vi "Open System.vi"(4 "Clear Previous Connections (False)":bool, 6 "ID Query (True)":bool=TRUE, 7 "IP Address":string, 8 "error in (no error)":errorcluster, 9 "Serial Configuration":T4={"Baud Rate"=9600, "Parity"=0, "Data Bits"=8, "Stop Bits"=10, "Flow Control"=0} {"Flow Control" items=["None", "XON/XOFF", "RTS/CTS", "XON/XOFF & RTS/CTS", "DTR/DSR", "XON/XOFF & DTR/DSR"]; "Stop Bits" items=["1.0"=10, "2.0"=20]; "Data Bits" items=["7"=7, "8"=8]; "Parity" items=["None", "Odd", "Even"]; "Baud Rate" items=["300"=300, "600"=600, "1200"=1200, "2400"=2400, "4800"=4800, "9600"=9600, "19200"=19200]}, 10 "Comms Layer":T2, 11 "VISA resource name":refnum<visa-resource-name>) -> (0 "error out":errorcluster, 1 "# of Instruments":i32, 2 "Serial Number(s)":string[](array[string]), 3 "Mercury Reference Out":T1, 5 "S/W Version(s)":string[](array[string]))   [LabVIEW 2018, in "Mercury iXX.lvlib" / "System.lvlib"]
doc: "Opens communication with a Mercury instrument on the chosen communication bus."
uses:
  System.lvlib
  Serial Settings.ctl
  Comms Transport Layer.ctl
  Mercury Reference.ctl
  Query Dynamic Reference.ctl
  Lookup Reference FGV Enum.ctl
  VISA Flush IO Buffer Mask.ctl
  Mercury iXX.lvlib
panel:
  in  "Reset (True)":bool=TRUE
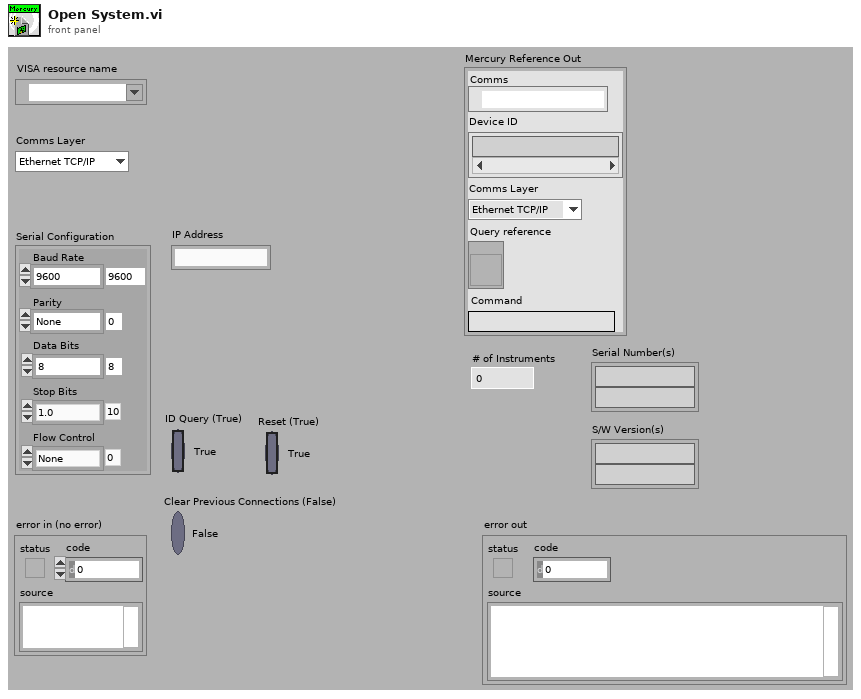
[diagram p1: front panel]
types:
  T1 = typedef "Mercury iXX.lvlib/Mercury Reference.ctl" = cluster{"Comms":refnum<visa-resource-name>, "Device ID":string[], "Comms Layer":T2, "Command":string, "Query reference":T3}
  T2 = typedef "Mercury iXX.lvlib/Comms Transport Layer.ctl" = enum16{"Ethernet TCP/IP", "USB", "ISOBus - RS-232", "GPIB"}
  T3 = typedef "Mercury iXX.lvlib/Query Dynamic Reference.ctl" = refnum<vi>
  T4 = typedef "Mercury iXX.lvlib/Serial Settings.ctl" = cluster{"Baud Rate":u32, "Parity":u16, "Data Bits":u16, "Stop Bits":u16, "Flow Control":u16}
  T5 = typedef "Mercury iXX.lvlib/Lookup Reference FGV Enum.ctl" = enum16{"Check VISA", "Get VI Ref", "Set VI ref", "Delete Single Ref", "Clear All"}
  T6 = typedef "VISA Flush IO Buffer Mask.ctl" = u16
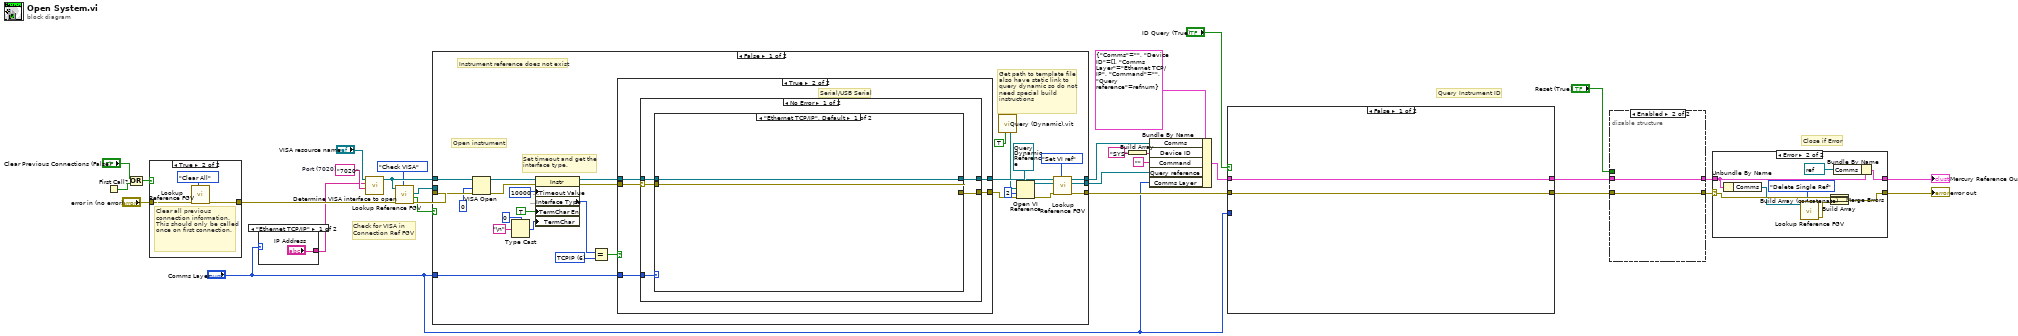
[diagram p0: block diagram]
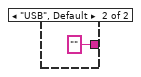
[diagram p2: hidden frame]
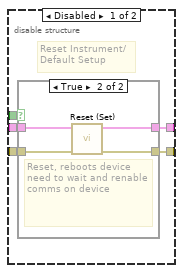
[diagram p4: hidden frame]
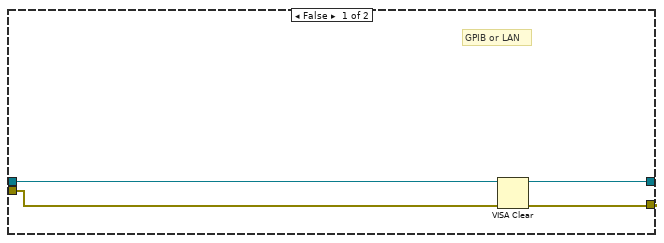
[diagram p6: hidden frame]
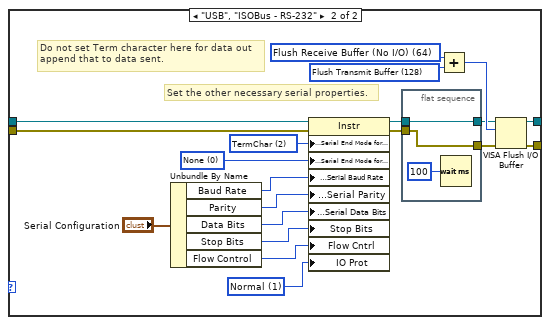
[diagram p7: hidden frame]
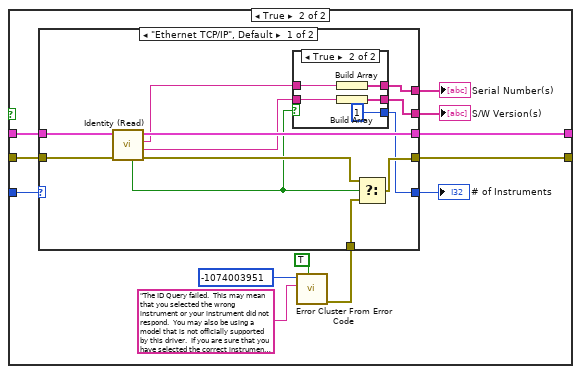
[diagram p11: hidden frame]
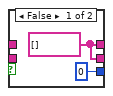
[diagram p12: hidden frame]
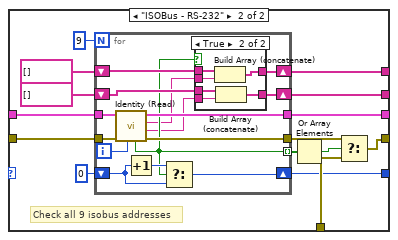
[diagram p13: hidden frame]
diagram:
  w30 = "7020"  # Port (7020)
  # "Check for VISA in \nConnection Ref FGV"
  # "Close if Error"
  # "Query Instrument ID"
  n1 = First Call?() -> (First Call?: T/F=w3:bool)
  n2 = Or(x="Clear Previous Connections (False)", y=w3) -> (x .or. y?=w4:bool)
  n3 = case shown="True" w4 {
    tunnel: "error in (no error)" -> [w31 w34]
    tunnel: [w31 w33] -> w5
    frame False {
    }
    frame True {
      # "Clear all previous connection information. This should only be called once on first connection."
      n4 = call "Lookup Reference FGV.vi"("State"=Lookup_Reference_FGV_Enum."Clear All", "error in"=w34) -> ("error out"=w33:errorcluster)  [unwired: 3 in, 6 out]
    }
  }
  n5 = case shown="\"Ethernet TCP/IP\"" "Comms Layer" {
    tunnel: ["IP Address" "" ("IP Address")] -> w1
    frame "Ethernet TCP/IP" {
    }
    frame "USB", Default {
    }
  }
  n6 = call "Determine VISA interface to open.vi"("Port (7020)"=w30, "IP Address"=w1, "VISA resource name"="VISA resource name") -> ("VISA resource name out"=w12:refnum<visa-resource-name>)  [unwired: 8 out]
  n7 = call "Lookup Reference FGV.vi"("State"=Lookup_Reference_FGV_Enum."Check VISA", "error in"=w5, "VISA In"=w12) -> ("error out"=w13:errorcluster, "Found Ref?"=w9:bool, "Query ref"=w8:T3)  [unwired: 2 in, 4 out]
  n8 = case shown="False" w9 {
    tunnel: w13 -> [w64 w108]
    tunnel: [w41 w108] -> w28
    tunnel: w12 -> [w54 w107]
    tunnel: [w43 w107] -> w16
    tunnel: "Comms Layer" -> [w49 _]
    tunnel: w8 -> [_ w106]
    tunnel: [w45 w106] -> w10
    frame False {
      w60 = u16 6 items=["GPIB"=1, "VXI"=2, "GPIB-VXI"=3, "Serial"=4, "PXI"=5, "TCPIP"=6, "USB"=7] ("Interface Information:Interface Type")
      # "Get path to template file\nalso have static link to \nquery dynamic so do not\nneed special build\ninstructions"
      # "Instrument reference does not exist"
      # "Set timeout and get the\ninterface type."
      # "Open instrument"
      n9 = VISA Open(access mode=u32 0, error in (no error)=w64, VISA resource name=w54) -> (VISA resource name=w58:refnum<visa-resource-name>, error out=w57:errorcluster)  [unwired: 2 out]
      n10 = Type Cast(type=u8 0 ("Message Based Settings:Termination Character"), x="\n") -> (*(type *) &x=w51:u8)
      n11 = property on="Property Node" class="Instr"(reference=w58, error in=w57, "General Settings:Timeout Value"=u32 10000, "TermChar En"=TRUE ("Message Based Settings:Termination Character Enable"), "TermChar"=w51) -> (reference out=w56:refnum<visa-resource-name>, error out=w55:errorcluster, "Interface Information:Interface Type"=w63:u16)
      n12 = Equal?(x=w63, y=w60) -> (x = y?=w61:bool)
      n13 = case shown="True" w61 {
        tunnel: [w66 w73] -> w44
        tunnel: [w65 w72] -> w47
        tunnel: w56 -> [w67 w71]
        tunnel: w55 -> [w68 w70]
        tunnel: w49 -> [_ w69]
        frame False {
          # "GPIB or LAN"
          n14 = VISA Clear(VISA resource name=w67, error in (no error)=w68) -> (VISA resource name out=w66:refnum<visa-resource-name>, error out=w65:errorcluster)
        }
        frame True {
          # "Serial/USB Serial"
          n15 = case shown="No Error" w70 {
            tunnel: w71 -> [w76 w105]
            selector: w70 -> [w75 w104]
            tunnel: [w78 w105] -> w73
            tunnel: [w77 w104] -> w72
            tunnel: w69 -> [w74 _]
            frame No Error {
              n16 = case shown="\"Ethernet TCP/IP\", Default" w74 {
                tunnel: [w80 w88] -> w78
                tunnel: [w79 w89] -> w77
                tunnel: w76 -> [w80 w90]
                tunnel: w75 -> [w79 w92]
                frame "Ethernet TCP/IP", Default {
                }
                frame "USB", "ISOBus - RS-232" {
                  w86 = T6 128 items=["Flush Receive Buffer"=16, "Write Transmit Buffer to Device"=32, "Flush Receive Buffer (No I/O)"=64, "Flush Transmit Buffer"=128] ("Mask")
                  w87 = T6 64 items=["Flush Receive Buffer"=16, "Write Transmit Buffer to Device"=32, "Flush Receive Buffer (No I/O)"=64, "Flush Transmit Buffer"=128] ("Mask")
                  w91 = u16 2 items=["None", "LastBit", "TermChar"] ("Serial Settings:Serial End Mode for Reads")
                  w100 = u16 1 items=["Normal"=1, "VXI/FDC"=2, "GPIB/HS488"=3, "Serial-TCPIP-USB/488 Strings"=4, "USBTMC/Vendor-Specific"=5] ("Message Based Settings:IO Protocol")
                  w95 = u16 0 items=["None", "LastBit", "TermChar"] ("Serial Settings:Serial End Mode for Reads")
                  # "Do not set Term character here for data out append that to data sent."
                  # "Set the other necessary serial properties."
                  n17 = Unbundle By Name("Serial Configuration") -> ("Baud Rate"=w97:u32, "Parity"=w99:u16, "Data Bits"=w98:u16, "Stop Bits"=w94:u16, "Flow Control"=w93:u16)
                  n18 = property on="Property Node" class="Instr"(reference=w90, error in=w92, "Serial Settings:Serial End Mode for Reads"=w91, "Serial Settings:Serial End Mode for Writes"=w95, "Serial Settings:Serial Baud Rate"=w97, "Serial Settings:Serial Parity"=w99, "Serial Settings:Serial Data Bits"=w98, "Stop Bits"=w94, "Flow Cntrl"=w93, "IO Prot"=w100) -> (reference out=w84:refnum<visa-resource-name>, error out=w82:errorcluster)
                  n19 = flat-sequence {
                    tunnel: w84 -> [w102]
                    tunnel: [w102] -> w83
                    tunnel: w82 -> [w101]
                    tunnel: [w101] -> w81
                    frame #0 {
                      n20 = Wait (ms)(milliseconds to wait=u32 100) -> ()  [unwired: 1 out]
                    }
                  }
                  n21 = Add(x=w87, y=w86) -> (x+y=w85:T6)
                  n22 = VISA Flush I/O Buffer(VISA resource name=w83, mask (16)=w85, error in (no error)=w81) -> (VISA resource name out=w88:refnum<visa-resource-name>, error out=w89:errorcluster)
                }
              }
            }
            frame Error {
              # "If there is an error in, do not attempt to set additional serial parameters."
            }
          }
        }
      }
      n23 = call "Query (Dynamic).vit"("Path Only"=TRUE) -> ("path"=w39:path)  [unwired: 5 in, 5 out]
      n24 = Open VI Reference(type specifier VI Refnum (for type only)=T3 refnum ("Query reference"), vi path=w39, options=2, error in (no error)=w47) -> (vi reference=w46:T3, error out=w42:errorcluster)  [unwired: 1 in, 1 out]
      n25 = call "Lookup Reference FGV.vi"("State"=Lookup_Reference_FGV_Enum."Set VI ref", "error in"=w42, "Query ref in"=w46, "VISA In"=w44) -> ("error out"=w41:errorcluster, "Query ref"=w45:T3, "VISA Out"=w43:refnum<visa-resource-name>)  [unwired: 1 in, 4 out]
    }
    frame True {
      # "Read connection ref from FGV"
      # "Instrument Reference Exists."
    }
  }
  n26 = Build Array("SYS") -> (w18:string[])
  n27 = Bundle By Name(cluster=T1 {"Comms"="", "Device ID"=[], "Comms Layer"=enum."Ethernet TCP/IP", "Command"="", "Query reference"=refnum} ("Mercury Reference"), "Comms"=w16, "Device ID"=w18, "Command"="", "Query reference"=w10, "Comms Layer"="Comms Layer") -> (w15:T1)
  n28 = case shown="False" "ID Query (True)" {
    tunnel: [w109 w122] -> w22
    tunnel: [w110 w119] -> w23
    tunnel: w15 -> [w110 w120]
    tunnel: w28 -> [w109 w121]
    tunnel: "Comms Layer" -> [_ w115]
    frame False {
    }
    frame True {
      n29 = call "Error Cluster From Error Code.vi"("show call chain? (False)"=TRUE, "error message (\"\")"="The ID Query failed.  This may mean that you selected the wrong instrument or your instrument did not respond.  You may also be using a model that is not officially supported by this driver.  If you are sure that you have selected the correct instrument and it is responding, try disabling the ID Query." ("Source (VI Name)"), "error code (0)"=-1074003951 ("Code")) -> ("error out"=w118:errorcluster)  [unwired: 1 in, 5 out]
      n30 = case shown="\"Ethernet TCP/IP\", Default" w115 {
        tunnel: [w134 w151] -> w122
        tunnel: w121 -> [w129 w155]
        tunnel: w120 -> [w132 w156]
        tunnel: [w131 w149] -> w119
        tunnel: w118 -> [w133 w153]
        tunnel: [w124 w144] -> w114
        tunnel: [w125 w143] -> w113
        tunnel: [w126 w142] -> w112
        frame "Ethernet TCP/IP", Default {
          n31 = call "Identity (Read).vi"("error in"=w129, "Mercury Reference In"=w132) -> ("error out"=w130:errorcluster, "S/W Version"=w127:string, "Serial Number"=w128:string, "Mercury Reference Out"=w131:T1, "Instrument Valid?"=w123:bool)  [unwired: 1 in, 4 out]
          n32 = case shown="True" w123 {
            tunnel: w128 -> [_ w141]
            tunnel: w127 -> [_ w140]
            tunnel: [w135 w139] -> w126
            tunnel: [w135 w138] -> w125
            tunnel: [0 1] -> w124
            frame False {
              w135 = string[] []
            }
            frame True {
              n33 = Build Array(w141) -> (w138:string[])
              n34 = Build Array(w140) -> (w139:string[])
            }
          }
          n35 = Select(t=w130, s=w123, f=w133) -> (s? t:f=w134:errorcluster)
        }
        frame "ISOBus - RS-232" {
          # "Check all 9 isobus addresses"
          n36 = for {
            N: 9 -> [_]
            tunnel: w156 -> [w171]
            tunnel: w155 -> [w170]
            tunnel: [w168] -> w152
            tunnel: [w159] -> w154 mode=indexing
            tunnel: [w167] -> w149
            shift-right: [w165] -> w144
            shift-left: 0 -> [w164]
            shift-right: [w160] -> w142
            shift-left: string[] [] -> [w161]
            shift-right: [w162] -> w143
            shift-left: string[] [] -> [w163]
            i -> [w169]
            n37 = call "Identity (Read).vi"("ISOBUS address"=w169, "error in"=w170, "Mercury Reference In"=w171) -> ("error out"=w168:errorcluster, "S/W Version"=w157:string, "Serial Number"=w158:string, "Mercury Reference Out"=w167:T1, "Instrument Valid?"=w159:bool)  [unwired: 4 out]
            n38 = Increment(x=w164) -> (x+1=w166:i32)
            n39 = Select(t=w166, s=w159, f=w164) -> (s? t:f=w165:i32)
            n40 = case shown="True" w159 {
              tunnel: w163 -> [w173 w179]
              tunnel: [w173 w178] -> w162
              tunnel: w161 -> [w172 w177]
              tunnel: [w172 w176] -> w160
              tunnel: w158 -> [_ w175]
              tunnel: w157 -> [_ w174]
              frame False {
              }
              frame True {
                n41 = Build Array (concatenate)(w179, w175) -> (w178:string[])
                n42 = Build Array (concatenate)(w177, w174) -> (w176:string[])
              }
            }
          }
          n43 = Or Array Elements(Boolean array=w154) -> (logical OR=w150:bool)
          n44 = Select(t=w152, s=w150, f=w153) -> (s? t:f=w151:errorcluster)
        }
      }
      "Serial Number(s)" <- w113
      "S/W Version(s)" <- w112
      "# of Instruments" <- w114
    }
  }
  n45 = disable-structure shown="Enabled" {
    disable-tunnel: "Reset (True)" -> [w184 _]
    disable-tunnel: [w183 w192] -> w25
    disable-tunnel: [w182 w191] -> w24
    disable-tunnel: w23 -> [w181 w192]
    disable-tunnel: w22 -> [w180 w191]
    frame Disabled {
      # "Reset Instrument/\nDefault Setup"
      n46 = case shown="True" w184 {
        tunnel: w180 -> [w186 w189]
        tunnel: [w186 w187] -> w182
        tunnel: w181 -> [w185 w190]
        tunnel: [w185 w188] -> w183
        frame False {
        }
        frame True {
          # "Reset, reboots device need to wait and renable comms on device"
          n47 = call "Reset (Set).vi"("error in"=w189, "Mercury Reference In"=w190) -> ("error out"=w187:errorcluster, "Mercury Reference Out"=w188:T1)  [unwired: 6 in, 2 out]
        }
      }
    }
    frame Enabled {
    }
  }
  n48 = case shown="Error" w24 {
    selector: w24 -> [w193 w204]
    tunnel: w25 -> [w194 w199]
    tunnel: [w194 w203] -> w14
    tunnel: [w193 w201] -> w21
    frame No Error {
    }
    frame Error {
      n49 = Unbundle By Name(w199) -> ("Comms"=w198:refnum<visa-resource-name>)
      n50 = call "Lookup Reference FGV.vi"("State"=Lookup_Reference_FGV_Enum."Delete Single Ref", "VISA In"=w198) -> ("error out"=w200:errorcluster)  [unwired: 3 in, 6 out]
      n51 = Build Array(w204, w200) -> (w196:errorcluster[])
      n52 = Build Array (concatenate)(w196) -> (w195:errorcluster[])
      n53 = Merge Errors(w195) -> (w201:errorcluster)
      n54 = Bundle By Name(cluster=w199, "Comms"=refnum<visa-resource-name> refnum ("VISA resource name out")) -> (w203:T1)
    }
  }
  "error out" <- w21
  "Mercury Reference Out" <- w14
